vi "solar_voy_def Export (Targets).vi"(8 "error in (no error)":errorcluster, 10 "ALL PACKETS":T1[](array[typedef]) {"last_time" format="%<%H:%M:%S%3u %m/%d/%y>T"}, 11 "CosmosDir":path) -> (0 "error out":errorcluster, 1 "First Registered Target":string, 2 "TARGETS":string[](array[string]), 3 "dup CosmosDir":path)   [LabVIEW 2018]
doc: "This exports the packets to the corresponding COSMOS target definition folders:\ncosmos\\config\\targets\\TARGET\\cmd_tlm\\TARGET_cmd|tlm.txt"
uses:
  solar_voy_def_ctl PATH.ctl
  solar_voy_def_ctl PACKET_ID.ctl
  solar_voy_def_ctl ITEM TYPE.ctl
  type/solar_type Item Type.ctl
  solar_voy_def_ctl ITEM.ctl
  solar_voy_def_ctl PACKET.ctl
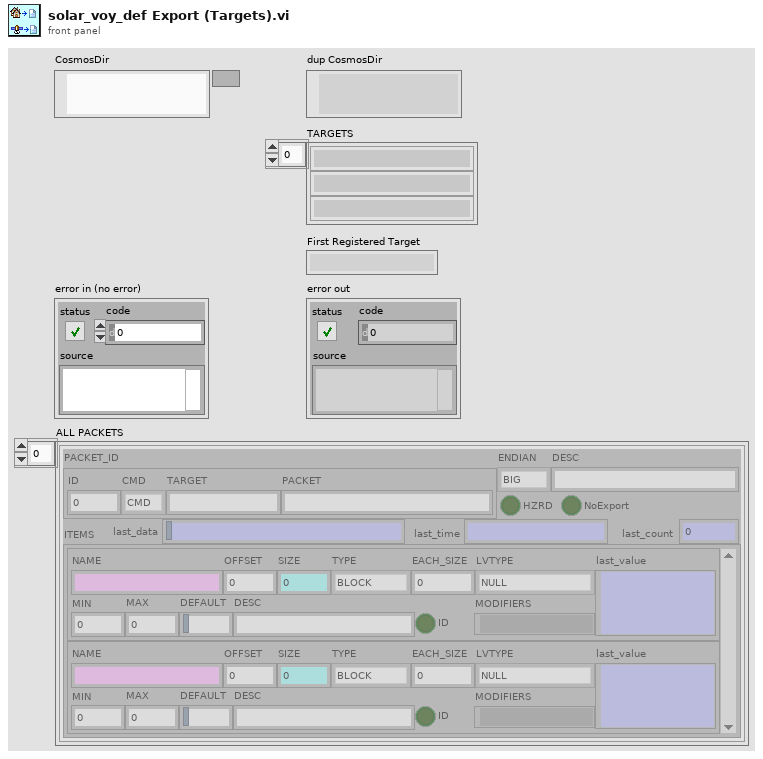
[diagram p1: front panel]
types:
  T1 = typedef "solar_voy_def_ctl PACKET.ctl" = cluster{"PACKET_ID":T2, "ENDIAN":enum8{"BIG", "LITTLE"}, "DESC":string, "HZRD":bool, "ITEMS":T3[], "NoExport":bool, "last_time":timestamp, "last_count":u32, "last_data":string}
  T2 = typedef "solar_voy_def_ctl PACKET_ID.ctl" = cluster{"ID":u16, "CMD":enum8{"CMD", "TLM"}, "TARGET":string, "PACKET":string}
  T3 = typedef "solar_voy_def_ctl ITEM.ctl" = cluster{"NAME":string, "OFFSET":i32, "SIZE":i32, "TYPE":T4, "EACH_SIZE":i32, "LVTYPE":T5, "MIN":dbl, "MAX":dbl, "DEFAULT":string, "DESC":string, "ID":bool, "MODIFIERS":variant, "last_value":variant}
  T4 = typedef "solar_voy_def_ctl ITEM TYPE.ctl" = enum8{"BLOCK", "INT", "UINT", "FLOAT", "STRING"}
  T5 = typedef "solar_type Item Type.ctl" = enum16{"NULL", "UNKNOWN", "CLUSTER", "I8", "I16", "I32", "I64", "U8", "U16", "U32", "U64", "U8_ENUM", "U16_ENUM", "U32_ENUM", "SGL", "DBL", "BOOLEAN", "STRING", "PATH", "VISA", "TAG", "TIME", "I8_1D", "I16_1D", "I32_1D", "I64_1D", "U8_1D", "U16_1D", "U32_1D", "U64_1D", "U8_ENUM_1D", "U16_ENUM_1D", "U32_ENUM_1D", "SGL_1D", "DBL_1D", "BOOLEAN_1D", "STRING_1D", "PATH_1D", "VISA_1D", "TAG_1D", "TIME_1D", "I8_2D", "I16_2D", "I32_2D", "I64_2D", "U8_2D", "U16_2D", "U32_2D", "U64_2D", "U8_ENUM_2D", "U16_ENUM_2D", "U32_ENUM_2D", "SGL_2D", "DBL_2D", "BOOLEAN_2D", "STRING_2D", "PATH_2D", "VISA_2D", "TAG_2D", "TIME_2D"}
  T6 = typedef "solar_voy_def_ctl PATH.ctl" = enum8{"..", "config", "config/data", "config/system", "config/targets", "config/targets/TARGET", "config/targets/TARGET/cmd_tlm", "config/targets/TARGET/lib", "config/targets/TARGET/screens", "config/tools", "config/tools/cmd_tlm_server", "config/tools/data_viewer", "config/tools/handbook_creator", "config/tools/launcher", "config/tools/limits_monitor", "config/tools/opengl_builder", "config/tools/script_runner", "config/tools/table_manager", "config/tools/test_runner", "config/tools/tlm_extractor", "config/tools/tlm_grapher", "config/tools/tlm_viewer", "lib", "outputs", "outputs/handbooks", "outputs/logs", "outputs/saved_config", "outputs/tables", "outputs/tmp", "procedures", "tools", "Launcher.bat", "config/system/system.txt", "config/targets/TARGET/cmd_tlm/TARGET_cmd.txt", "config/targets/TARGET/cmd_tlm/TARGET_tlm.txt", "config/targets/TARGET/cmd_tlm_server.txt", "config/targets/TARGET/target.txt", "config/tools/cmd_tlm_server/cmd_tlm_server.txt", "config/tools/data_viewer/data_viewer.txt", "config/tools/handbook_creator/handbook_creator.txt", "config/tools/launcher/launcher.txt", "config/tools/limits_monitor/limits_monitor.txt", "config/tools/opengl_builder/opengl_builder.txt", "config/tools/script_runner/script_runner.txt", "config/tools/table_manager/table_manager.txt", "config/tools/test_runner/test_runner.txt", "config/tools/tlm_extractor/tlm_extractor.txt", "config/tools/tlm_grapher/tlm_grapher.txt", "config/tools/tlm_viewer/tlm_viewer.txt"}
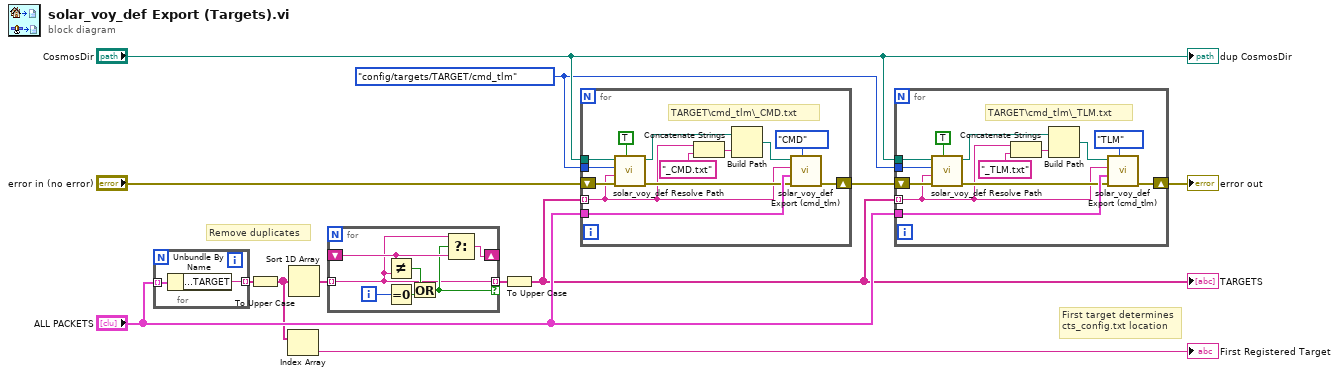
[diagram p0: block diagram]
diagram:
  w7 = solar_voy_def_ctl_PATH."config/targets/TARGET/cmd_tlm" ("PATH (..=Root)")
  # "First target determines\ncts_config.txt location"
  # "Remove duplicates"
  n1 = for {
    tunnel: "ALL PACKETS" -> [w14] mode=indexing
    tunnel: [w13] -> w10 mode=indexing
    n2 = Unbundle By Name(w14) -> ("PACKET_ID.TARGET"=w13:string)
  }
  n3 = To Upper Case(1:w10) -> (0:w2:string[])
  n4 = Index Array(array=w2) -> (element=→"First Registered Target":string)  [unwired: 1 in]
  n5 = Sort 1D Array(array=w2) -> (sorted array=w11:string[])
  n6 = for {
    tunnel: w11 -> [w15] mode=indexing
    tunnel: [w15] -> w6 mode=indexing if=w16
    shift-right: [w18] -> _
    shift-left: _ -> [w17]
    i -> [w21]
    n7 = Not Equal?(x=w17, y=w15) -> (x != y?=w19:bool)
    n8 = Equal To 0?(x=w21) -> (x = 0?=w20:bool)
    n9 = Or(x=w19, y=w20) -> (x .or. y?=w16:bool)
    n10 = Select(t=w15, s=w16, f=w17) -> (s? t:f=w18:string)
  }
  n11 = To Upper Case(1:w6) -> (0:w4:string[])
  "TARGETS" <- w4
  n12 = for {
    tunnel: "CosmosDir" -> [w30]
    shift-right: [w34] -> w9
    shift-left: "error in (no error)" -> [w29]
    tunnel: "ALL PACKETS" -> [w33]
    tunnel: w4 -> [w22] mode=indexing
    tunnel: w7 -> [w27]
    # "TARGET\\cmd_tlm\\_CMD.txt"
    n13 = call "solar_voy_def Resolve Path.vi"("Create Folder? (T)"=TRUE, "error in (no error)"=w29, "TARGET"=w22, "PATH (..=Root)"=w27, "COSMOS_ROOT"=w30) -> ("error out"=w28:errorcluster, "Resolved Path"=w24:path)  [unwired: 5 in]
    n14 = Concatenate Strings(w22, "_CMD.txt" ("string")) -> (w25:string)
    n15 = Build Path(base path=w24, name or relative path=w25) -> (appended path=w23:path)
    n16 = call "solar_voy_def Export (cmd_tlm).vi"("CMD"=enum8{"CMD", "TLM"}."CMD", "error in (no error)"=w28, "ALL PACKETS"=w33, "Target Name"=w22, "cmd_tlm.txt in"=w23) -> ("error out"=w34:errorcluster)  [unwired: 5 in, 1 out]
  }
  n17 = for {
    tunnel: "CosmosDir" -> [w43]
    shift-right: [w47] -> w3
    shift-left: w9 -> [w42]
    tunnel: "ALL PACKETS" -> [w46]
    tunnel: w4 -> [w35] mode=indexing
    tunnel: w7 -> [w40]
    # "TARGET\\cmd_tlm\\_TLM.txt"
    n18 = call "solar_voy_def Resolve Path.vi"("Create Folder? (T)"=TRUE, "error in (no error)"=w42, "TARGET"=w35, "PATH (..=Root)"=w40, "COSMOS_ROOT"=w43) -> ("error out"=w41:errorcluster, "Resolved Path"=w37:path)  [unwired: 5 in]
    n19 = Concatenate Strings(w35, "_TLM.txt" ("string")) -> (w38:string)
    n20 = Build Path(base path=w37, name or relative path=w38) -> (appended path=w36:path)
    n21 = call "solar_voy_def Export (cmd_tlm).vi"("CMD"=enum8{"CMD", "TLM"}."TLM", "error in (no error)"=w41, "ALL PACKETS"=w46, "Target Name"=w35, "cmd_tlm.txt in"=w36) -> ("error out"=w47:errorcluster)  [unwired: 5 in, 1 out]
  }
  "error out" <- w3
  "dup CosmosDir" <- "CosmosDir"
